vi "String Indicator BG Color.vi"(10 "BG Color":u32(colorbox), 11 "Ex Event Actor in":refnum<class "Ex Event Actor.lvclass">) -> (0 "error out":errorcluster)   [LabVIEW 2021, in "Ex Event Actor.lvlib" / "Ex Event Actor.lvclass"]
uses:
  Ex Event Actor.lvclass
  Ex Event Actor.lvclass/Ex Event Actor.ctl
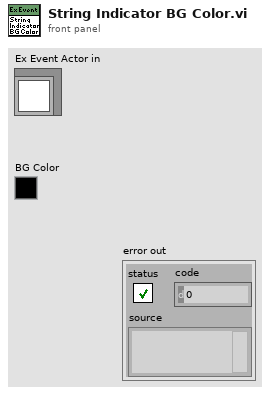
[diagram p1: front panel]
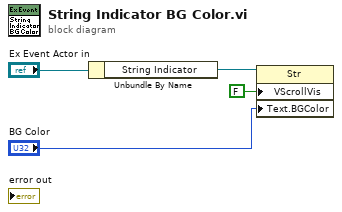
[diagram p0: block diagram]
diagram:
  n1 = Unbundle By Name("Ex Event Actor in") -> ("String Indicator"=w3:refnum<vi>)
  n2 = property class="Str"(reference=w3, "VScrollVis"=FALSE ("Vertical Scrollbar Visible"), "Text.BGColor"="BG Color") -> ()  [unwired: 1 in, 2 out]
